vi "Status DAQmx.vi"(8 "error in (no error)":errorcluster, 10 "data":variant, 11 "Control-Client in":refnum<class "Control-Client.lvclass">) -> (0 "error out":errorcluster, 2 "error IO":errorcluster, 3 "Control-Client out":refnum<class "Control-Client.lvclass">)   [LabVIEW 2015, in "Control-Client.lvclass"]
uses:
  Control-Client.lvclass
  dependecies/ControlsVIs/Clusters-def/Commands-CLIENT.ctl
  dependecies/ControlsVIs/Clusters-def/Message types.ctl
  dependecies/ControlsVIs/Clusters-def/DAQmx-Reply-Connect-client.ctl
  Control-Client.lvclass/Control-Client.ctl
  dependecies/XControls/CellsDL/ControlDL.xctl
  controls/Gauge_pump/Gauge_pump.xctl
  DAQmxTasks/DAQmxTaskContainer/DAQmxTaskContainer.lvclass
  Message/Message.lvclass
  GeneralFunctionality/GeneralFunctionality.lvclass
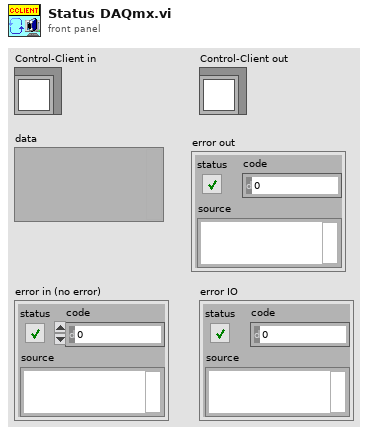
[diagram p1: front panel]
types:
  T1 = typedef "DAQmxTaskContainer.lvclass/DAQmx-Reply-Connect-client.ctl" = cluster{"on/off":bool, "RelayKeyHeater/off":bool, "LaserShutter":bool, "AcceleratorShutter":bool, "Power":bool, "Faraday Cup Status":bool, "error":errorcluster}
  T2 = typedef "Message types.ctl" = string
  T3 = typedef "Control-Client.lvclass/Commands-CLIENT.ctl" = string
  T4 = typedef "Control-Client.lvclass/Controls-with-permissions_CLIENT.ctl" = cluster{"Server ON/OFF":refnum<vi>, "Detector connect":refnum<vi>, "DL connect":refnum<vi>, "DAQmx connect":refnum<vi>, "All connect":refnum<vi>, "Start measurement":refnum<vi>, "Move Crystal":refnum<vi>, "Relay key heater":refnum<vi>, "Laser Shutter":refnum<vi>, "Accelerator Shutter":refnum<vi>, "Power":refnum<vi>, "Unlock":refnum<vi>, "RT":refnum<vi>, "Faraday Cup":refnum<vi>, "Osc connect":refnum<vi>, "ELYSE pulses":refnum<vi>, "Cells":refnum<vi>, "ControlDL":refnum<vi>, "Pump":refnum<vi>, "# par point":refnum<vi>, "Alarm":refnum<vi>, "oscilloscopeRead":refnum<vi>, "WCM_state":refnum<vi>}
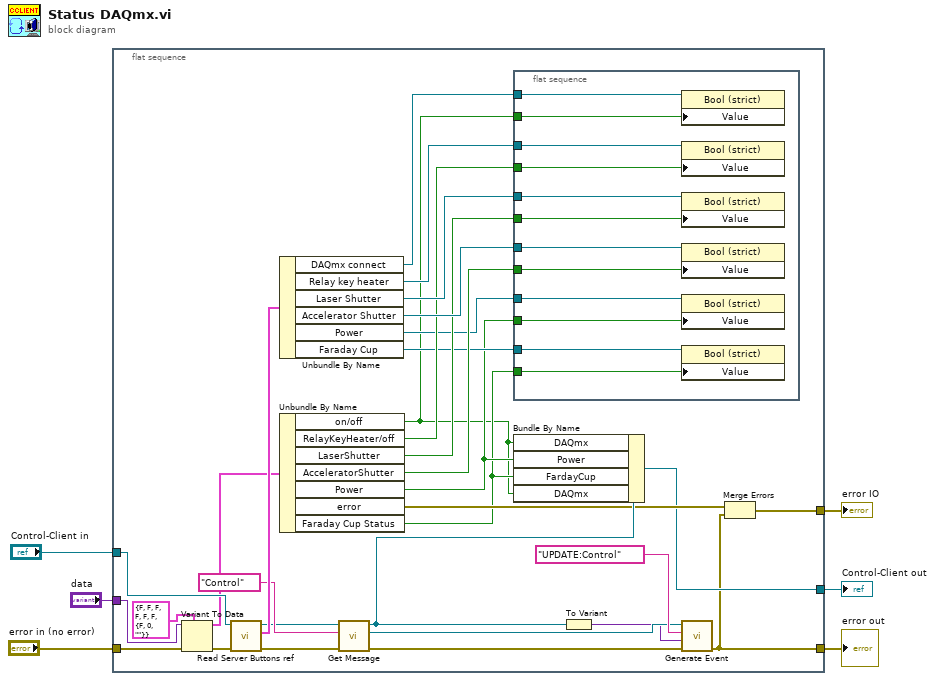
[diagram p0: block diagram]
diagram:
  n1 = flat-sequence {
    tunnel: "data" -> [w37]
    tunnel: "Control-Client in" -> [w36]
    tunnel: "error in (no error)" -> [w34]
    tunnel: [w10] -> w5
    tunnel: [w23] -> w6
    tunnel: [w8] -> w1
    frame #0 {
      n2 = Variant To Data(error in=w34, type=T1 {"on/off"=FALSE, "RelayKeyHeater/off"=FALSE, "LaserShutter"=FALSE, "AcceleratorShutter"=FALSE, "Power"=FALSE, "Faraday Cup Status"=FALSE, "error"={"status"=FALSE, "code"=0, "source"=""}} ("output cluster"), Variant=w37) -> (data=w24:T1, error out=w35:errorcluster)
      n3 = call "Read Server Buttons ref.vi"("error in (no error)"=w35, "Control-Client in"=w36) -> ("error out"=w25:errorcluster, "Server Buttons ref"=w33:T4, "Control-Client out"=w26:refnum<class "Control-Client.lvclass">)  [unwired: 7 in]
      n4 = Unbundle By Name(w33) -> ("DAQmx connect"=w32:refnum<vi>, "Relay key heater"=w20:refnum<vi>, "Laser Shutter"=w19:refnum<vi>, "Accelerator Shutter"=w18:refnum<vi>, "Power"=w13:refnum<vi>, "Faraday Cup"=w12:refnum<vi>)
      n5 = Unbundle By Name(w24) -> ("on/off"=w7:bool, "RelayKeyHeater/off"=w16:bool, "LaserShutter"=w15:bool, "AcceleratorShutter"=w14:bool, "Power"=w11:bool, "error"=w17:errorcluster, "Faraday Cup Status"=w9:bool)
      n6 = call "Get Message.vi"("error in (no error)"=w25, "Message type"=T2 "Control", "GeneralFunctionality en entrée"=w26) -> ("error out"=w28:errorcluster, "Message.lvclass"=w30:refnum<class "Message.lvclass">, "GeneralFunctionality en sortie"=w22:refnum<class "Control-Client.lvclass">)  [unwired: 6 in]
      n7 = flat-sequence {
        tunnel: w32 -> [w49]
        tunnel: w7 -> [w48]
        tunnel: w20 -> [w47]
        tunnel: w19 -> [w46]
        tunnel: w18 -> [w45]
        tunnel: w16 -> [w44]
        tunnel: w15 -> [w43]
        tunnel: w14 -> [w42]
        tunnel: w13 -> [w41]
        tunnel: w12 -> [w40]
        tunnel: w11 -> [w39]
        tunnel: w9 -> [w38]
        frame #0 {
          n8 = property class="Bool (strict)"(reference=w49, "Value"=w48) -> ()  [unwired: 1 in, 2 out]
          n9 = property class="Bool (strict)"(reference=w47, "Value"=w44) -> ()  [unwired: 1 in, 2 out]
          n10 = property class="Bool (strict)"(reference=w46, "Value"=w43) -> ()  [unwired: 1 in, 2 out]
          n11 = property class="Bool (strict)"(reference=w45, "Value"=w42) -> ()  [unwired: 1 in, 2 out]
          n12 = property class="Bool (strict)"(reference=w41, "Value"=w39) -> ()  [unwired: 1 in, 2 out]
          n13 = property class="Bool (strict)"(reference=w40, "Value"=w38) -> ()  [unwired: 1 in, 2 out]
        }
      }
      n14 = Bundle By Name(cluster=w22, "DAQmx"=w7, "Power"=w11, "FardayCup"=w9, "DAQmx"=w7) -> (w10:refnum<class "Control-Client.lvclass">)
      n15 = To Variant(anything=w22) -> (Variant=w27:variant)
      n16 = call "Generate Event.vi"("error in (no error)"=w28, "Data"=w27, "Command"=T3 "UPDATE:Control" ("Commands-Client"), "Message en entrée"=w30) -> ("error out"=w8:errorcluster)  [unwired: 6 in, 1 out]
      n17 = Merge Errors(w17, w8) -> (w23:errorcluster)
    }
  }
  "error IO" <- w6
  "Control-Client out" <- w5
  "error out" <- w1
